vi "Insert Pannel Template.vi"(8 "error in":errorcluster caption="错误输入（无错误）", 9 "Split Mode":T1, 11 "PanelDataNode in":refnum<class "PanelDataNode.lvclass"> caption="DNL_LabVIEW Object in") -> (0 "error out":errorcluster caption="错误输出", 3 "PanelDataNode out":refnum<class "PanelDataNode.lvclass"> caption="DNL_LabVIEW Object out")   [LabVIEW 2016, in "PanelDataNode.lvclass"]
uses:
  PanelDataNode.lvclass
  C:/Users/CL/Desktop/ZcDAQprj0811/ZcDAQprj/Modules/DAQ-Display/PanelSplitToolkit/PanelLinkNode/PanelLinkNode.lvclass
  Split Mode.ctl
  PanelLinkNode/PanelLinkNode.lvclass/PanelLinkNode.ctl
  PanelDataNode.lvclass/PanelDataNode.ctl
  PanelObject/PanelObject.lvclass
  PanelLinkNode/PanelLinkNode.lvclass
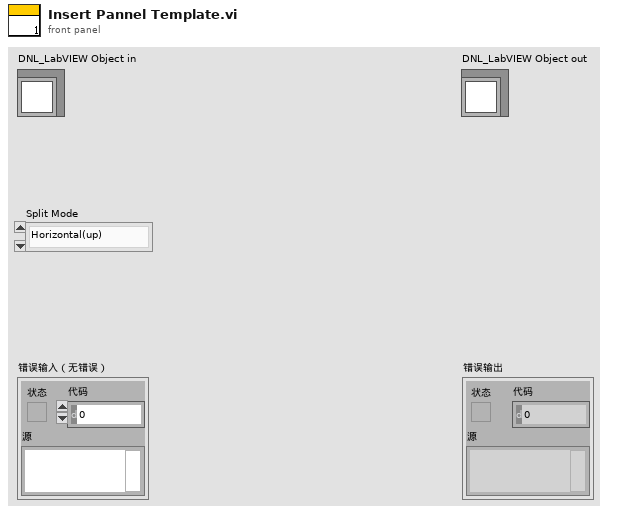
[diagram p1: front panel]
types:
  T1 = typedef "PanelDataNode.lvclass/Split Mode.ctl" = enum16{"Horizontal(up)", "Vertical(left)", "Horizontal(down)", "Vertical(right)"}
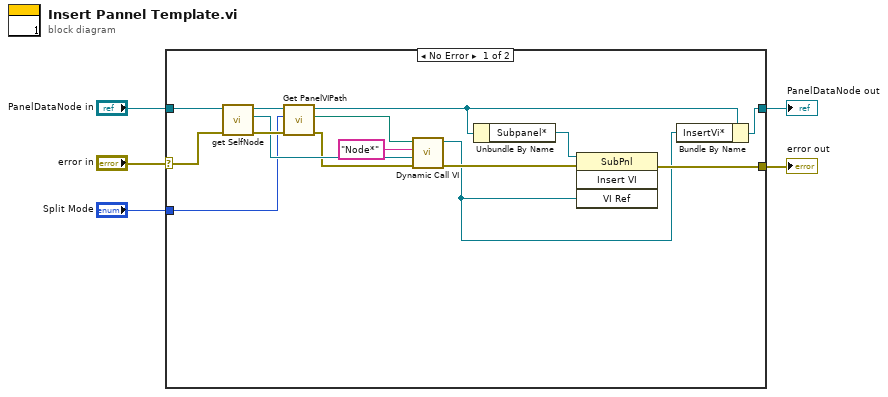
[diagram p0: block diagram]
diagram:
  n1 = case shown="No Error" "error in" {
    selector: "error in" -> [w7 w22]
    tunnel: [w11 w22] -> w4
    tunnel: [w8 w21] -> w2
    tunnel: "PanelDataNode in" -> [w18 w21]
    tunnel: "Split Mode" -> [w6 _]
    frame No Error {
      n2 = call "get SelfNode.vi"("error in (no error)"=w7, "PanelLinkNode输入"=w18) -> ("error out"=w16:errorcluster, "SelfNode*"=w15:refnum<data-value>, "PanelLinkNode输出"=w17:refnum<class "PanelDataNode.lvclass">)  [unwired: 7 in]
      n3 = call-dynamic "Get PanelVIPath.vi"("error in (no error)"=w16, "Split Mode"=w6, "PanelDataNode 输入"=w17) -> ("error out"=w13:errorcluster, "panel path"=w20:path, "PanelDataNode 输出"=w10:refnum<class "PanelDataNode.lvclass">)  [unwired: 4 in]
      n4 = call "Dynamic Call VI.vi"("error in"=w13, "CtrlValue"=w15, "CtrlName"="Node*" ("控件名"), "Vi Path"=w20) -> ("错误输出"=w12:errorcluster, "vi reference"=w9:refnum<vi>)  [unwired: 6 in]
      n5 = Unbundle By Name(w10) -> ("Subpanel*"=w14:refnum<vi>)
      n6 = invoke class="SubPnl" method="Insert VI"(reference=w14, error in=w12, "VI Ref"=w9) -> (error out=w11:errorcluster)  [unwired: 1 in, 3 out]
      n7 = Bundle By Name(cluster=w10, "InsertVi*"=w9) -> (w8:refnum<class "PanelDataNode.lvclass">)
    }
    frame Error {
    }
  }
  "error out" <- w4
  "PanelDataNode out" <- w2
